vi "Write String 1.vi"(8 "error in (no error)":errorcluster, 10 "String 1":string="myString", 11 "Section 2 in":refnum<class "Section 2.lvclass">) -> (0 "error out":errorcluster, 3 "Section 2 out":refnum<class "Section 2.lvclass">)   [LabVIEW 2016, in "LVOOP Introduction.lvlib" / "Section 2.lvclass"]
uses:
  Section 2.lvclass
  Section 2.lvclass/Section 2.ctl
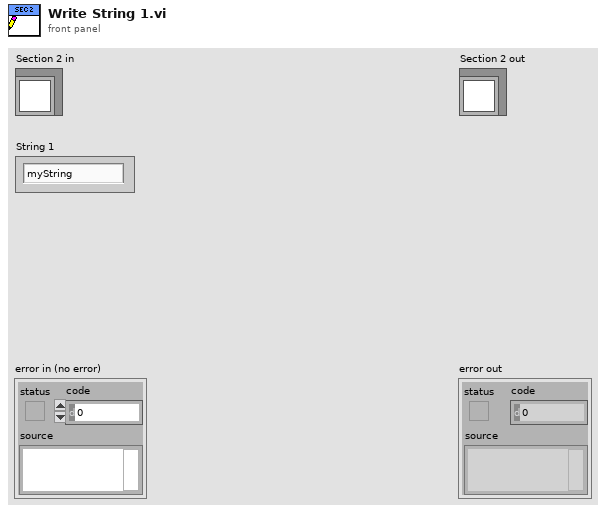
[diagram p1: front panel]
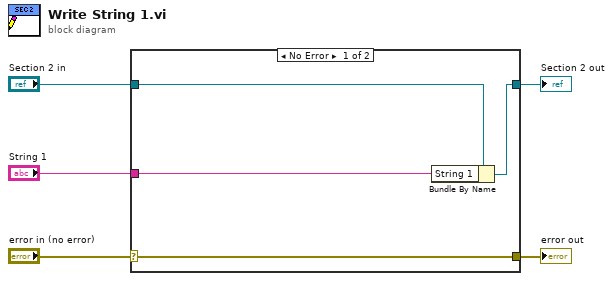
[diagram p0: block diagram]
diagram:
  n1 = case shown="No Error" "error in (no error)" {
    selector: "error in (no error)" -> [w9 w10]
    tunnel: [w9 w10] -> w4
    tunnel: [w7 w11] -> w2
    tunnel: "Section 2 in" -> [w8 w11]
    tunnel: "String 1" -> [w6 _]
    frame No Error {
      n2 = Bundle By Name(cluster=w8, "String 1"=w6) -> (w7:refnum<class "Section 2.lvclass">)
    }
    frame Error {
    }
  }
  "error out" <- w4
  "Section 2 out" <- w2
